vi "WaveMove.vi"(0 "Length":dbl, 1 "Spacing":dbl, 2 "LineNo":i32, 3 "error in":errorcluster, 4 "MinJT":dbl, 5 "Vel":dbl, 6 "MaxJT":dbl, 7 "StartPos":dbl[](array[numeric]), 8 "Acc":dbl, 9 "Direction":enum16{"Y to X", "X to Y"}(ring)) -> (10 "error out":errorcluster)   [LabVIEW 2022 SP3]
uses:
  Global 3.vi
  Newport.XPS.CommandInterface
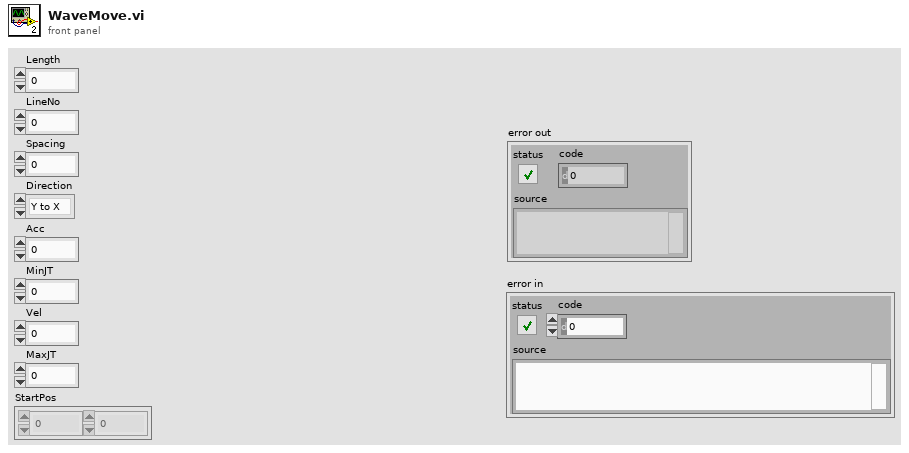
[diagram p1: front panel]
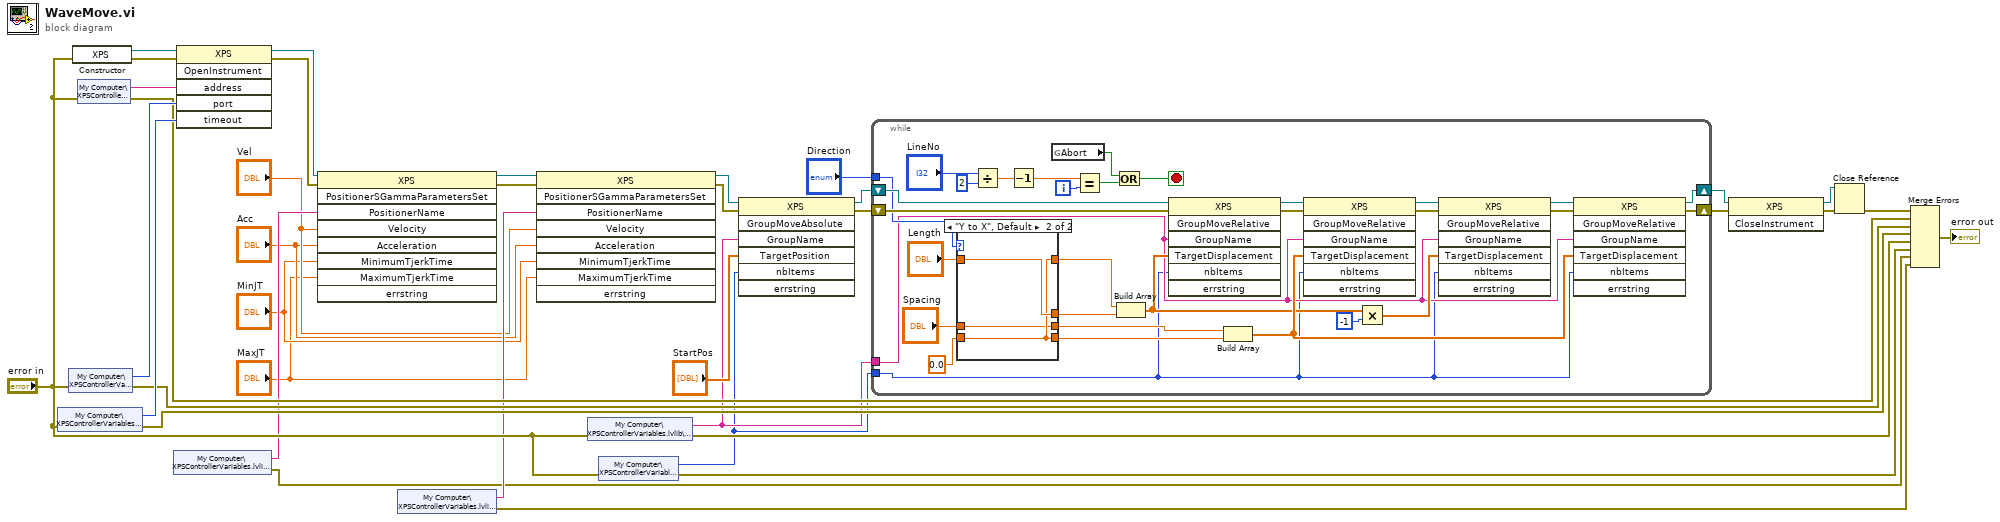
[diagram p0: block diagram]
diagram:
  n1 = shared-variable "My Computer\\XPSControllerVariables.lvlib\\Timeout"(error in="error in") -> (w33:i16, error out=w28:errorcluster)
  n2 = shared-variable "My Computer\\XPSControllerVariables.lvlib\\Port"(error in="error in") -> (w34:i16, error out=w29:errorcluster)
  n3 = constructor class="XPS"(error in="error in") -> (reference out=w37:refnum<k24>, error out=w36:errorcluster)  [unwired: 2 in, 1 out]
  n4 = shared-variable "My Computer\\XPSControllerVariables.lvlib\\IP"(error in="error in") -> (w35:string, error out=w30:errorcluster)
  n5 = shared-variable "My Computer\\XPSControllerVariables.lvlib\\PosNameX"() -> (w16:string, error out=w9:errorcluster)  [unwired: 1 in]
  n6 = invoke class="XPS" method="OpenInstrument"(reference=w37, error in=w36, "address"=w35, "port"=w34, "timeout"=w33) -> (reference out=w22:refnum<k24>, error out=w21:errorcluster)  [unwired: 1 in, 4 out]
  n7 = invoke class="XPS" method="PositionerSGammaParametersSet"(reference=w22, error in=w21, "PositionerName"=w16, "Velocity"="Vel", "Acceleration"="Acc", "MinimumTjerkTime"="MinJT", "MaximumTjerkTime"="MaxJT") -> (reference out=w20:refnum<k24>, error out=w19:errorcluster)  [unwired: 2 in, 7 out]
  n8 = shared-variable "My Computer\\XPSControllerVariables.lvlib\\PosNameY"() -> (w15:string, error out=w8:errorcluster)  [unwired: 1 in]
  n9 = invoke class="XPS" method="PositionerSGammaParametersSet"(reference=w20, error in=w19, "PositionerName"=w15, "Velocity"="Vel", "Acceleration"="Acc", "MinimumTjerkTime"="MinJT", "MaximumTjerkTime"="MaxJT") -> (reference out=w18:refnum<k24>, error out=w17:errorcluster)  [unwired: 2 in, 7 out]
  n10 = shared-variable "My Computer\\XPSControllerVariables.lvlib\\GroupName"(error in="error in") -> (w3:string, error out=w27:errorcluster)
  n11 = shared-variable "My Computer\\XPSControllerVariables.lvlib\\nbitem"(error in="error in") -> (w2:i16, error out=w23:errorcluster)
  n12 = invoke class="XPS" method="GroupMoveAbsolute"(reference=w18, error in=w17, "GroupName"=w3, "TargetPosition"="StartPos", "nbItems"=w2) -> (reference out=w7:refnum<k24>, error out=w6:errorcluster)  [unwired: 2 in, 5 out]
  n13 = while {
    tunnel: w3 -> [w42]
    tunnel: w2 -> [w41]
    shift-right: [w48] -> w5
    shift-left: w7 -> [w69]
    shift-right: [w47] -> w4
    shift-left: w6 -> [w68]
    tunnel: "Direction" -> [w53]
    i -> [w64]
    stop <- w61 stop-if-true
    n14 = case shown="\"Y to X\", Default" w53 {
      tunnel: [w72 w74] -> w60
      tunnel: "Length" -> [w72 w75]
      tunnel: [w71 w75] -> w58
      tunnel: 0.0 -> [w71 w74]
      tunnel: [w71 w73] -> w56
      tunnel: [w70 w74] -> w55
      tunnel: "Spacing" -> [w70 w73]
      frame "X to Y" {
      }
      frame "Y to X", Default {
      }
    }
    n15 = Divide(x="LineNo", y=2) -> (x/y=w38:dbl)
    n16 = Decrement(x=w38) -> (x-1=w65:dbl)
    n17 = global read "Global 3.vi" "Abort"() -> (w63:bool)
    n18 = Equal?(x=w65, y=w64) -> (x = y?=w62:bool)
    n19 = Or(x=w63, y=w62) -> (x .or. y?=w61:bool)
    n20 = Build Array(w60, w58) -> (w45:dbl[])
    n21 = invoke class="XPS" method="GroupMoveRelative"(reference=w69, error in=w68, "GroupName"=w42, "TargetDisplacement"=w45, "nbItems"=w41) -> (reference out=w67:refnum<k24>, error out=w66:errorcluster)  [unwired: 2 in, 5 out]
    n22 = Build Array(w56, w55) -> (w46:dbl[])
    n23 = invoke class="XPS" method="GroupMoveRelative"(reference=w67, error in=w66, "GroupName"=w42, "TargetDisplacement"=w46, "nbItems"=w41) -> (reference out=w52:refnum<k24>, error out=w51:errorcluster)  [unwired: 2 in, 5 out]
    n24 = Multiply(x=w45, y=-1) -> (x*y=w43:dbl[])
    n25 = invoke class="XPS" method="GroupMoveRelative"(reference=w52, error in=w51, "GroupName"=w42, "TargetDisplacement"=w43, "nbItems"=w41) -> (reference out=w50:refnum<k24>, error out=w49:errorcluster)  [unwired: 2 in, 5 out]
    n26 = invoke class="XPS" method="GroupMoveRelative"(reference=w50, error in=w49, "GroupName"=w42, "TargetDisplacement"=w46, "nbItems"=w41) -> (reference out=w48:refnum<k24>, error out=w47:errorcluster)  [unwired: 2 in, 5 out]
  }
  n27 = invoke class="XPS" method="CloseInstrument"(reference=w5, error in=w4) -> (reference out=w32:refnum<k24>, error out=w31:errorcluster)  [unwired: 1 in, 1 out]
  n28 = Close Reference(reference=w32, error in (no error)=w31) -> (error out=w26:errorcluster)
  n29 = Merge Errors(w26, w30, w29, w28, w27, w23, w9, w8) -> (→"error out":errorcluster)
